vi "IMAQ ROI to MSC Image ROI.vi"(0 "IMAQ ROI Descriptor":T5 {"Contours"."Type" items=["No Selection", "Point", "Line", "Rectangle", "Oval", "Polygon", "Freehand Region", "Annulus", "Unused2", "Unused3", "Broken Line", "Freehand Line", "Rotated Rectangle"]}, 11 "error in":errorcluster) -> (4 "ROIs":T1[](array[typedef]) {"Type" items=["Point", "Line", "Rectangle", "Oval", "Freehand / Polygon"]}, 15 "error out":errorcluster)   [LabVIEW 2014]
doc: "Converts an IMAQ ROI Descriptor to MSC ROIs\n\n<B>Currently supported:</B>\n- Point\n- Line\n- Rectangle\n- Oval\n- Polygon\n- Freehand Region"
uses:
  MSC Image_class/controls/ROI.ctl
  MSC Image_class/controls/ROI Type.ctl
  MSC Image_class/controls/Contour.ctl
  MSC Image_class/controls/Contour hierarchy.ctl
  MSC Image_class/MSC Image.lvclass
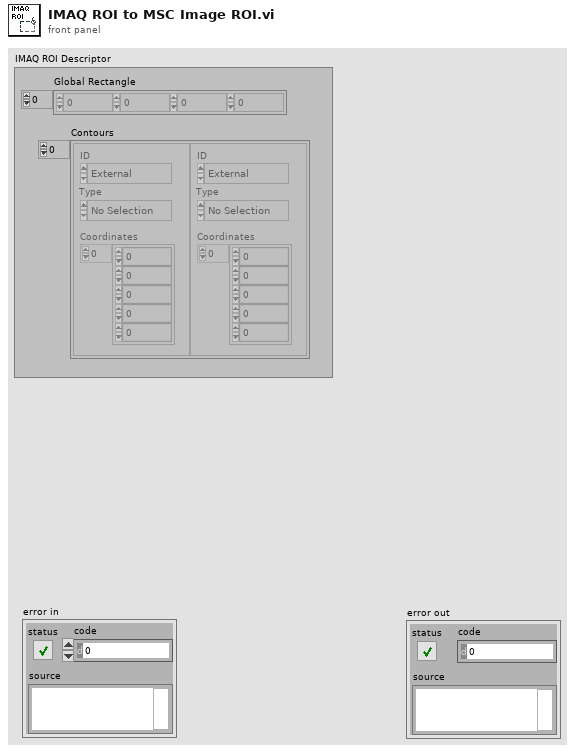
[diagram p1: front panel]
types:
  T1 = typedef "MSC Image.lvclass/ROI.ctl" = cluster{"Type":T2, "Parameters":dbl[], "Contour":T3, "Bounding Box":T3, "Contour Length":dbl, "ROI Area":dbl, "ROI Mean":dbl, "ROI Standard Deviation":dbl, "ROI Min":dbl, "ROI Max":dbl, "Hierarchy":T4, "Variant":variant, "Timestamp":timestamp}
  T2 = typedef "MSC Image.lvclass/ROI Type.ctl" = u16
  T3 = typedef "MSC Image.lvclass/Contour.ctl" = cluster{"x":i16, "y":i16}[]
  T4 = typedef "MSC Image.lvclass/Contour hierarchy.ctl" = cluster{"parent ID":i32, "children IDs":dbl[], "level":i32}
  T5 = typedef "ROI Descriptor" = cluster{"Global Rectangle":i32[], "Contours":cluster{"ID":enum32{"External", "Internal"}, "Type":u32, "Coordinates":i32[]}[]}
  T6 = cluster{"ID":enum32{"External", "Internal"}, "Type":u32, "Coordinates":i32[]}[]
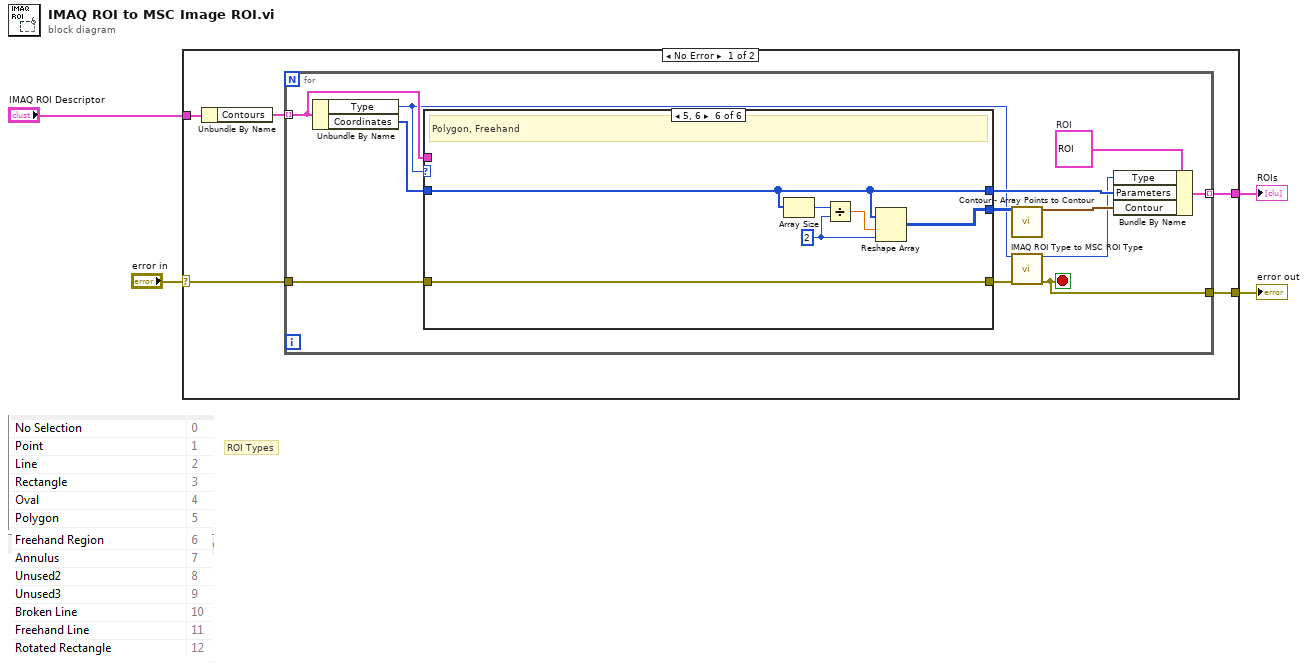
[diagram p0: block diagram]
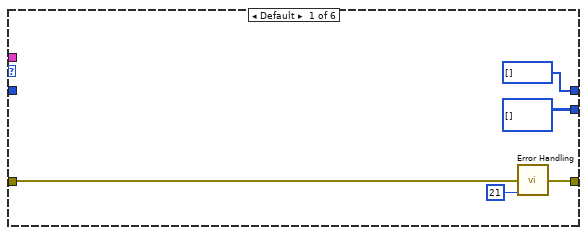
[diagram p2: hidden frame]
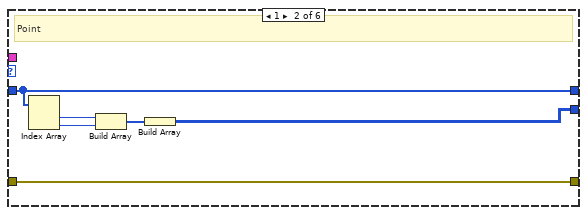
[diagram p3: hidden frame]
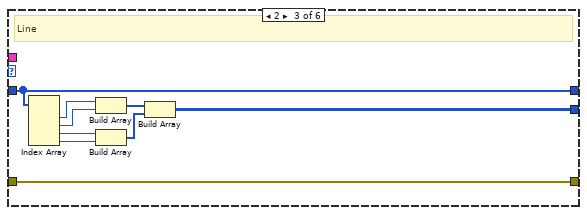
[diagram p4: hidden frame]
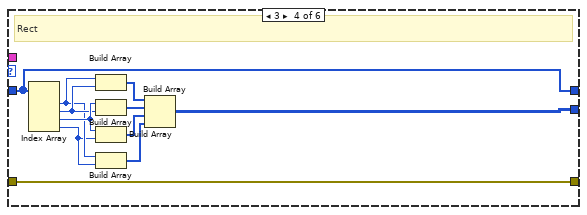
[diagram p5: hidden frame]
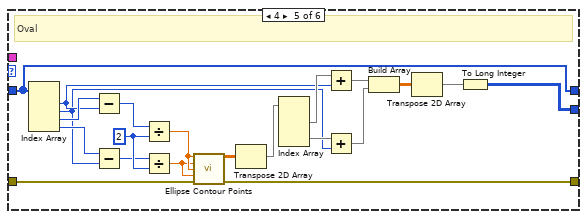
[diagram p6: hidden frame]
diagram:
  # "ROI Types"
  n1 = case shown="No Error" "error in" {
    selector: "error in" -> [w6 w80]
    tunnel: "IMAQ ROI Descriptor" -> [w9 _]
    tunnel: [w7 w80] -> w3
    tunnel: [w5 _] -> w1
    frame No Error {
      n2 = Unbundle By Name(w9) -> ("Contours"=w8:T6)
      n3 = for {
        tunnel: w8 -> [w20] mode=indexing
        tunnel: w6 -> [w19]
        tunnel: [w10] -> w7
        tunnel: [w14] -> w5 mode=indexing
        stop <- w10 stop-if-true
        w18 = T1 {"Type"=0, "Parameters"=[], "Contour"=[], "Bounding Box"=[], "Contour Length"=0.0, "ROI Area"=0.0, "ROI Mean"=0.0, "ROI Standard Deviation"=0.0, "ROI Min"=0.0, "ROI Max"=0.0, "Hierarchy"={"parent ID"=0, "children IDs"=[], "level"=0}, "Variant"=variant, "Timestamp"=timestamp(0 s since 1904-01-01)}  # ROI
        n4 = Unbundle By Name(w20) -> ("Type"=w13:u32, "Coordinates"=w21:i32[])
        n5 = case shown="5, 6" w13 {
          tunnel: w21 -> [_ w27 w33 w42 w53 w74]
          tunnel: [i32[][] [] w30 w37 w52 w66 w76] -> w16
          tunnel: w20 -> [_ _ _ _ _ _]
          tunnel: w19 -> [w22 w29 w36 w48 w70 w75]
          tunnel: [w23 w29 w36 w48 w69 w75] -> w11
          tunnel: [i32[] [] ("Coordinates") w27 w33 w42 w53 w74] -> w17
          frame Default {
            n6 = call "Error Handling.vi"("error in (no error)"=w22, "return type"=21 ("code")) -> ("error out"=w23:errorcluster)  [unwired: 12 in, 1 out]
          }
          frame 1 {
            # "Point"
            n7 = Index Array(array=w27) -> (element #1=w32:i32, element #2=w31:i32)  [unwired: 2 in]
            n8 = Build Array(w32, w31) -> (w28:i32[])
            n9 = Build Array(w28) -> (w30:i32[][])
          }
          frame 2 {
            # "Line"
            n10 = Index Array(array=w33) -> (element #1=w41:i32, element #2=w40:i32, element #3=w39:i32, element #4=w38:i32)  [unwired: 4 in]
            n11 = Build Array(w41, w40) -> (w35:i32[])
            n12 = Build Array(w39, w38) -> (w34:i32[])
            n13 = Build Array(w35, w34) -> (w37:i32[][])
          }
          frame 3 {
            # "Rect"
            n14 = Index Array(array=w42) -> (element #1=w45:i32, element #2=w46:i32, element #3=w47:i32, element #4=w44:i32)  [unwired: 4 in]
            n15 = Build Array(w45, w46) -> (w43:i32[])
            n16 = Build Array(w47, w46) -> (w51:i32[])
            n17 = Build Array(w47, w44) -> (w50:i32[])
            n18 = Build Array(w45, w44) -> (w49:i32[])
            n19 = Build Array(w43, w51, w50, w49) -> (w52:i32[][])
          }
          frame 4 {
            w71 = 2 ("y")
            # "Oval"
            n20 = Index Array(array=w53) -> (element #1=w56:i32, element #2=w55:i32, element #3=w73:i32, element #4=w72:i32)  [unwired: 4 in]
            n21 = Subtract(x=w73, y=w56) -> (x-y=w61:i32)
            n22 = Subtract(x=w72, y=w55) -> (x-y=w54:i32)
            n23 = Divide(x=w61, y=w71) -> (x/y=w68:dbl)
            n24 = Divide(x=w54, y=w71) -> (x/y=w67:dbl)
            n25 = call "Ellipse Contour Points.vi"("A"=w68, "B"=w67, "x-Shift"=w68, "y-shift"=w67, "error in"=w70) -> ("Contour Array Points"=w64:dbl[][], "error out"=w69:errorcluster)  [unwired: 9 in]
            n26 = Transpose 2D Array(2D array=w64) -> (transposed array=w65:dbl[][])
            n27 = Index Array(array=w65) -> (element #1=w62:dbl[], element #2=w63:dbl[])  [unwired: 4 in]
            n28 = Add(x=w62, y=w56) -> (x+y=w60:dbl[])
            n29 = Add(x=w63, y=w55) -> (x+y=w59:dbl[])
            n30 = Build Array(w60, w59) -> (w58:dbl[][])
            n31 = Transpose 2D Array(2D array=w58) -> (transposed array=w57:dbl[][])
            n32 = To Long Integer(number=w57) -> (32bit integer=w66:i32[][])
          }
          frame 5, 6 {
            w78 = 2 ("dimension size")
            # "Polygon, Freehand"
            n33 = Array Size(array=w74) -> (size(s)=w77:i32)
            n34 = Divide(x=w77, y=w78) -> (x/y=w79:dbl)
            n35 = Reshape Array(w74, w79, w78) -> (w76:i32[][])
          }
        }
        n36 = call "Contour - Array Points to Contour.vi"("Array Points"=w16) -> ("Contour"=w15:T3)  [unwired: 14 in]
        n37 = call "IMAQ ROI Type to MSC ROI Type.vi"("IMAQ ROI Type"=w13, "error in (no error)"=w11) -> ("MSC ROI Type"=w12:T2, "error out"=w10:errorcluster)  [unwired: 12 in]
        n38 = Bundle By Name(cluster=w18, "Type"=w12, "Parameters"=w17, "Contour"=w15) -> (w14:T1)
      }
    }
    frame Error {
    }
  }
  "error out" <- w3
  "ROIs" <- w1
